vi "autoNameFile.vi"(1 "num":dbl, 2 "File Basename":string, 3 "Folder Name":path=path "D:/users/marc/20180122_LiIon_EL/Freezing02/OutputHighT002p2.dat") -> (0 "path":path)   [LabVIEW 2011]
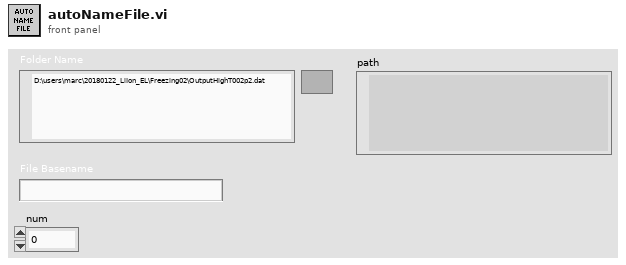
[diagram p1: front panel]
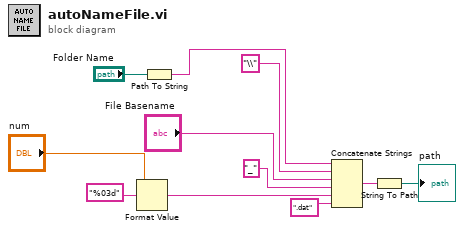
[diagram p0: block diagram]
diagram:
  n1 = Format Value(format string="%03d", value (0)="num") -> (output string=w9:string)  [unwired: 1 in]
  n2 = Path To String(path="Folder Name") -> (string=w10:string)
  n3 = Concatenate Strings(w10, "\\" ("string"), "File Basename", "_" ("string"), w9, ".dat" ("string")) -> (w7:string)
  n4 = String To Path(string=w7) -> (path=→"path":path)
